vi "InitStepper.vi"(8 "error in (no error)":errorcluster, 9 "RevSteps":u16, 10 "index(0/1)":i32, 11 "StepperMotor in":refnum<class "StepperMotor.lvclass">) -> (0 "error out":errorcluster, 3 "StepperMotor out":refnum<class "StepperMotor.lvclass">)   [LabVIEW 2022 SP3, in "Motorshield.lvlib" / "StepperMotor.lvclass"]
uses:
  StepperMotor.lvclass
  StepperMotor.lvclass/StepperMotor.ctl
  Motorshield/Motorshield.lvclass
  C:/Users/Carlos/Desktop/onlab/source/Motorshield/Motorshield/Motorshield.lvclass
  C:/Users/Carlos/Desktop/onlab/source/Motorshield/StepperMotor/StepperMotor.lvclass
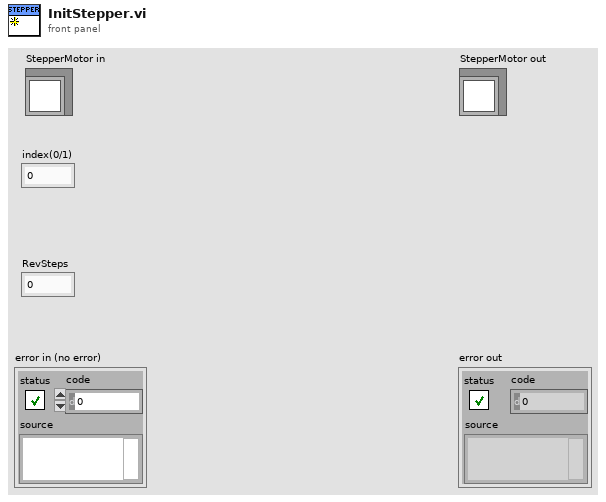
[diagram p1: front panel]
types:
  T1 = typedef "Motorshield.lvlib/StepperMotor.lvclass/StepperInfo.ctl" = cluster{"PWMA":u8, "AIn1pin":u8, "AIn2pin":u8, "PWMB":u8, "BIn1pin":u8, "BIn2pin 2":u8}
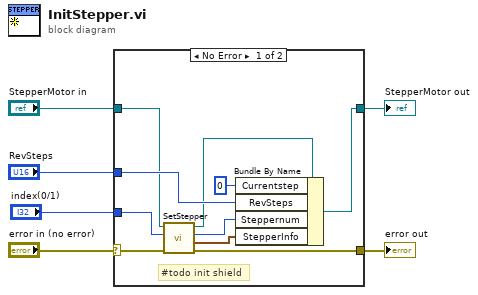
[diagram p0: block diagram]
diagram:
  n1 = case shown="No Error" "error in (no error)" {
    selector: "error in (no error)" -> [w14 w18]
    tunnel: [w13 w18] -> w5
    tunnel: [w16 w17] -> w3
    tunnel: "StepperMotor in" -> [w11 w17]
    tunnel: "RevSteps" -> [w15 _]
    tunnel: "index(0/1)" -> [w12 _]
    frame No Error {
      # "#todo init shield"
      n2 = call "SetStepper.vi"("error in (no error)"=w14, "index(0/1)"=w12, "Motorshield in"=w11) -> ("error out"=w13:errorcluster, "StepperInfo"=w9:T1, "index"=w8:i32, "Motorshield out"=w10:refnum<class "StepperMotor.lvclass">)  [unwired: 5 in]
      n3 = Bundle By Name(cluster=w10, "Currentstep"=u8 0, "RevSteps"=w15, "Steppernum"=w8, "StepperInfo"=w9) -> (w16:refnum<class "StepperMotor.lvclass">)
    }
    frame Error {
    }
  }
  "error out" <- w5
  "StepperMotor out" <- w3
